vi "Waveform to X,Y.vi"(4 "offset":dbl, 6 "Y":dbl[](array[numeric]), 7 "dx":dbl) -> (1 "Y":dbl[](array[numeric]), 2 "X":dbl[](array[numeric]))   [LabVIEW 2020]
uses:
  Math VIs/LinSpace (x0-dx-npts).vi
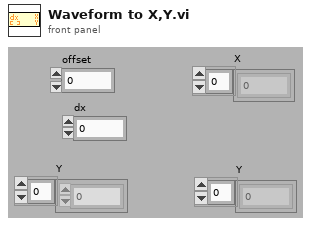
[diagram p1: front panel]
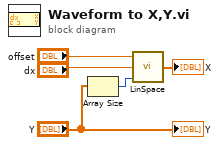
[diagram p0: block diagram]
diagram:
  n1 = Array Size(array="Y") -> (size(s)=w2:i32)
  n2 = call-poly "LinSpace.vi"("npts"=w2, "dx"="dx", "x0"="offset") -> ("Array"=→"X":dbl[])  [unwired: 1 in, 1 out]
  "Y" <- "Y"
